vi "data insert core.vi"(8 "error in (no error)":errorcluster, 9 "column information":T1[](array[typedef]), 10 "data":variant[](array[variant]), 11 "table":string) -> (0 "error out":errorcluster)   [LabVIEW 2016, in "斯坦道原位多参数.lvlib"]
uses:
  <vilib>/addons/database/Auxilliary.llb/DB Tools Column Info.ctl
  <vilib>/addons/database/Auxilliary.llb/DB Tools DataTypes.ctl
  <vilib>/Utility/sysdir.llb/System Directory Type.ctl
  <vilib>/addons/database/Auxilliary.llb/DB Tools Transaction.ctl
  <vilib>/addons/database/Auxilliary.llb/DB Tools Isolation Level.ctl
  <vilib>/addons/database/Auxilliary.llb/DB Tools Parameter Info.ctl
  <vilib>/addons/database/Auxilliary.llb/DB Tools Parameter Dir.ctl
  <vilib>/addons/database/Connection.llb/DB Tools Open Connec (String).vi
  <vilib>/addons/database/Connection.llb/Conn Transaction.vi
  <vilib>/addons/database/Connection.llb/Conn Execute.vi
  <vilib>/addons/database/Recordset.llb/Rec Destroy - Connection.vi
  <vilib>/addons/database/Command.llb/Cmd Set Parameter Value (C).vi
  <vilib>/addons/database/Auxilliary.llb/DB Tools Format Datetime String (Time Stamp).vi
  <vilib>/addons/database/Command.llb/Cmd Execute.vi
  <vilib>/addons/database/Recordset.llb/Rec Destroy - Command.vi
  <vilib>/addons/database/Command.llb/Cmd Delete.vi
  <vilib>/addons/database/NI_Database_API.lvlib
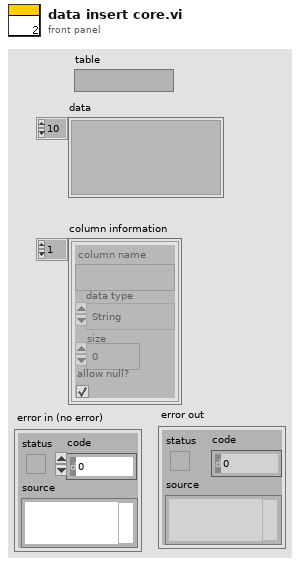
[diagram p1: front panel]
types:
  T1 = typedef "NI_Database_API.lvlib/DB Tools Column Info.ctl" = cluster{"column name":string, "data type":T2, "size":i32, "allow null?":bool}
  T2 = typedef "NI_Database_API.lvlib/DB Tools DataTypes.ctl" = enum16{"String", "Long (I32)", "Single (SGL)", "Double (DBL)", "Date/Time", "Binary"}
  T3 = typedef "NI_Database_API.lvlib/DB Tools Isolation Level.ctl" = enum16{"chaos", "read uncommitted", "read committed", "repeatable read", "serializable"}
  T4 = typedef "NI_Database_API.lvlib/DB Tools Transaction.ctl" = enum16{"begin", "commit", "rollback"}
  T5 = typedef "System Directory Type.ctl" = i32
  T6 = typedef "NI_Database_API.lvlib/Conn ObjectReference.ctl" = refnum<k1>
  T7 = typedef "NI_Database_API.lvlib/DB Tools Parameter Info.ctl" = cluster{"parameter name":string, "type":T2, "direction":T8, "value":variant}
  T8 = typedef "NI_Database_API.lvlib/DB Tools Parameter Dir.ctl" = enum32{"Input", "Output", "Input/Output", "Return Value"}
  T9 = typedef "NI_Database_API.lvlib/Rec ObjectReference.ctl" = refnum<k1>
  T10 = typedef "NI_Database_API.lvlib/Cmd ObjectReference.ctl" = refnum<k1>
  T11 = typedef "NI_Database_API.lvlib/Cmd-Rec Object Reference.ctl" = refnum<k1>
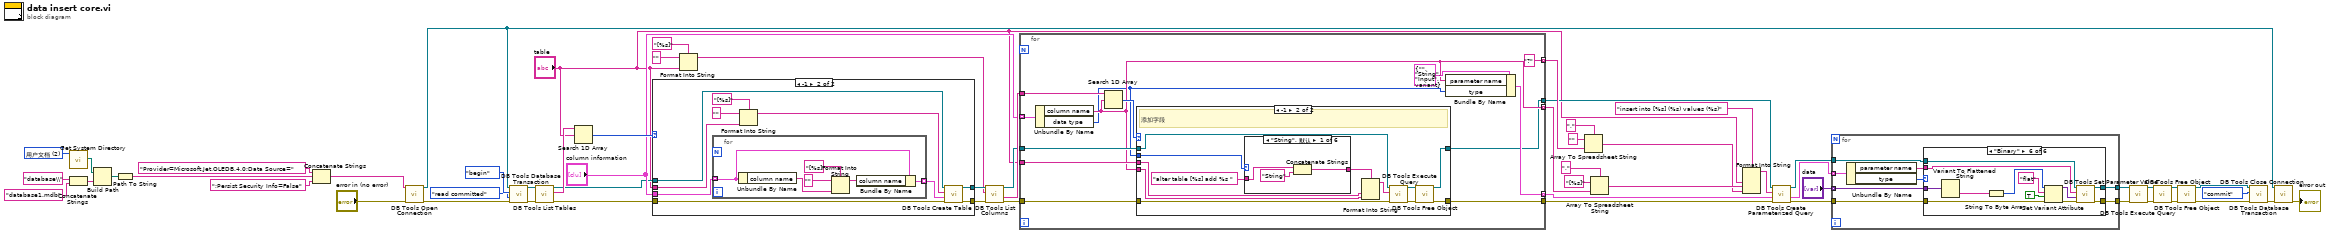
[diagram p0: block diagram]
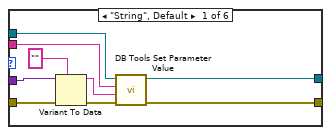
[diagram p2: hidden frame]
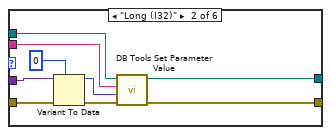
[diagram p3: hidden frame]
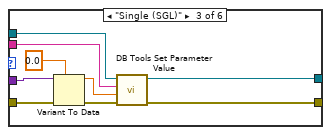
[diagram p4: hidden frame]
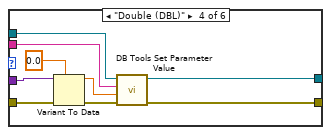
[diagram p5: hidden frame]
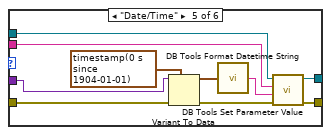
[diagram p6: hidden frame]
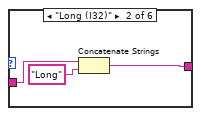
[diagram p8: hidden frame]
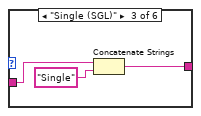
[diagram p9: hidden frame]
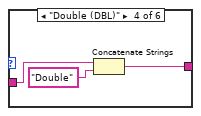
[diagram p10: hidden frame]
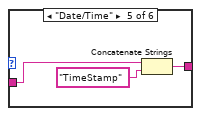
[diagram p11: hidden frame]
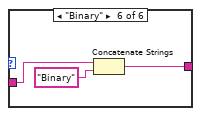
[diagram p12: hidden frame]
diagram:
  w59 = T5 2 items=["用户目录"=0, "用户桌面"=1, "用户文档"=2, "用户应用程序数据"=3, "用户设置"=4, "用户临时目录"=5, "公共文档"=6, "公共应用程序数据"=7, "公共设置"=8, "公共缓存"=13, "系统核心库"=9, "系统安装库"=10, "应用程序文件"=11, "启动盘根目录"=12] ("system directory type")
  n1 = call <vilib>:"Get System Directory.vi"("system directory type"=w59) -> ("system directory"=w57:path)  [unwired: 10 in]
  n2 = Concatenate Strings("database\\" ("condition"), "database1.mdb" ("database")) -> (w51:string)
  n3 = Build Path(base path=w57, name or relative path=w51) -> (appended path=w56:path)
  n4 = Path To String(path=w56) -> (string=w55:string)
  n5 = Concatenate Strings("Provider=Microsoft.Jet.OLEDB.4.0;Data Source=" ("condition"), w55, ";Persist Security Info=False" ("condition")) -> (w53:string)
  n6 = call-poly <vilib>:"DB Tools Open Connection.vi"("error in (no error)"="error in (no error)", "connection information"=w53) -> ("error out"=w13:errorcluster, "connection reference"=w5:T6)  [unwired: 6 in]
  n7 = call-poly <vilib>:"DB Tools Database Transaction.vi"("error in (no error)"=w13, "isolation level (chaos)"=DB_Tools_Isolation_Level."read committed", "operation (begin)"=DB_Tools_Transaction."begin", "connection reference"=w5) -> ("error out"=w12:errorcluster, "connection reference out"=w14:T6)  [unwired: 2 in]
  n8 = call <vilib>:"DB Tools List Tables.vi"("error in (no error)"=w12, "connection reference"=w14) -> ("error out"=w42:errorcluster, "tables"=w44:string[], "connection reference out"=w8:T6)  [unwired: 3 in]
  n9 = Search 1D Array(1D array=w44, element="table") -> (index of element=w43:i32)  [unwired: 1 in]
  n10 = case shown="-1" w43 {
    tunnel: w8 -> [w61 w71]
    tunnel: w42 -> [w60 w70]
    tunnel: "table" -> [_ w63]
    tunnel: "column information" -> [_ w67]
    tunnel: [w61 w69] -> w38
    tunnel: [w60 w68] -> w37
    frame 0, Default {
    }
    frame -1 {
      n11 = for {
        tunnel: w67 -> [w73] mode=indexing
        tunnel: [w72] -> w66 mode=indexing
        n12 = Unbundle By Name(w73) -> ("column name"=w77:string)
        n13 = Format Into String(format string="[%s]" ("格式字符串"), initial string="" ("初始字符串"), w77) -> (resulting string=w74:string)  [unwired: 1 in, 1 out]
        n14 = Bundle By Name(cluster=w73, "column name"=w74) -> (w72:T1)
      }
      n15 = Format Into String(format string="[%s]" ("格式字符串"), initial string="" ("初始字符串"), w63) -> (resulting string=w62:string)  [unwired: 1 in, 1 out]
      n16 = call <vilib>:"DB Tools Create Table.vi"("error in (no error)"=w70, "column information"=w66, "table"=w62, "connection reference"=w71) -> ("error out"=w68:errorcluster, "connection reference out"=w69:T6)  [unwired: 4 in]
    }
  }
  n17 = Format Into String(format string="[%s]" ("格式字符串"), initial string="" ("初始字符串"), "table") -> (resulting string=w1:string)  [unwired: 1 in, 1 out]
  n18 = call <vilib>:"DB Tools List Columns.vi"("error in (no error)"=w37, "table"=w1, "connection reference"=w38) -> ("error out"=w40:errorcluster, "columns"=w41:string[], "connection reference out"=w10:T6)  [unwired: 1 in, 1 out]
  n19 = for {
    tunnel: w10 -> [w88]
    tunnel: w41 -> [w90]
    tunnel: w40 -> [w87]
    tunnel: [w86] -> w36
    tunnel: "table" -> [w85]
    tunnel: "column information" -> [w84] mode=indexing
    tunnel: [w82] -> w35 mode=indexing
    tunnel: [w81] -> w29 mode=indexing
    tunnel: ["?"] -> w27 mode=indexing
    tunnel: [w78] -> w7
    n20 = Unbundle By Name(w84) -> ("column name"=w81:string, "data type"=w79:T2)
    n21 = Search 1D Array(1D array=w90, element=w81) -> (index of element=w89:i32)  [unwired: 1 in]
    n22 = case shown="-1" w89 {
      tunnel: [w92 w101] -> w86
      tunnel: w88 -> [w91 w100]
      tunnel: w81 -> [_ w99]
      tunnel: w87 -> [w92 w98]
      tunnel: w85 -> [_ w97]
      tunnel: w79 -> [_ w95]
      tunnel: [w91 w93] -> w78
      frame 0, Default {
      }
      frame -1 {
        # "添加字段"
        n23 = case shown="\"String\", 默认" w95 {
          tunnel: "alter table [%s] add %s " -> [w107 w110 w113 w116 w119 w122]
          tunnel: [w106 w109 w112 w115 w118 w121] -> w94
          frame "String", Default {
            n24 = Concatenate Strings(w107, "String" ("字符串")) -> (w106:string)
          }
          frame "Long (I32)" {
            n25 = Concatenate Strings(w110, "Long" ("字符串")) -> (w109:string)
          }
          frame "Single (SGL)" {
            n26 = Concatenate Strings(w113, "Single" ("字符串")) -> (w112:string)
          }
          frame "Double (DBL)" {
            n27 = Concatenate Strings(w116, "Double" ("字符串")) -> (w115:string)
          }
          frame "Date/Time" {
            n28 = Concatenate Strings(w119, "TimeStamp" ("字符串")) -> (w118:string)
          }
          frame "Binary" {
            n29 = Concatenate Strings(w122, "Binary" ("字符串")) -> (w121:string)
          }
        }
        n30 = Format Into String(format string=w94, w97, w99) -> (resulting string=w102:string)  [unwired: 2 in, 1 out]
        n31 = call-poly <vilib>:"DB Tools Execute Query.vi"("error in (no error)"=w98, "SQL query"=w102, "connection reference"=w100) -> ("error out"=w103:errorcluster, "recordset reference"=w104:T9)  [unwired: 5 in]
        n32 = call-poly <vilib>:"DB Tools Free Object.vi"("error in (no error)"=w103, "recordset reference"=w104) -> ("error out"=w101:errorcluster, "connection reference"=w93:T6)  [unwired: 8 in]
      }
    }
    n33 = Bundle By Name(cluster=T7 {"parameter name"="", "type"=enum."String", "direction"=enum."Input", "value"=variant} ("parameter information"), "parameter name"=w81, "type"=w79) -> (w82:T7)
  }
  n34 = Array To Spreadsheet String(delimiter (Tab)="," ("分隔符(Tab)"), array=w27, 3:"" ("格式字符串")) -> (spreadsheet string=w26:string)
  n35 = Array To Spreadsheet String(delimiter (Tab)="," ("分隔符(Tab)"), array=w29, 3:"[%s]" ("格式字符串")) -> (spreadsheet string=w28:string)
  n36 = Format Into String(format string="insert into [%s] (%s) values (%s)" ("格式字符串"), "table", w28, w26) -> (resulting string=w25:string)  [unwired: 2 in, 1 out]
  n37 = call <vilib>:"DB Tools Create Parameterized Query.vi"("error in (no error)"=w36, "parameters"=w35, "SQL query"=w25, "connection reference"=w7) -> ("error out"=w24:errorcluster, "parameters out"=w23:T7[], "command reference"=w9:T10)  [unwired: 3 in]
  n38 = for {
    tunnel: w9 -> [w127]
    tunnel: w24 -> [w125]
    tunnel: w23 -> [w130] mode=indexing
    tunnel: "data" -> [w128] mode=indexing
    tunnel: [w124] -> w6
    tunnel: [w123] -> w22
    n39 = Unbundle By Name(w130) -> ("parameter name"=w126:string, "type"=w129:T2)
    n40 = case shown="\"Binary\"" w129 {
      tunnel: w128 -> [w134 w142 w149 w159 w176 w180]
      tunnel: w127 -> [w137 w146 w153 w163 w174 w188]
      tunnel: w126 -> [w136 w145 w152 w158 w173 w187]
      tunnel: w125 -> [w131 w140 w150 w160 w171 w179]
      tunnel: [w133 w144 w154 w162 w170 w186] -> w124
      tunnel: [w132 w143 w151 w161 w169 w185] -> w123
      frame "String", Default {
        n41 = Variant To Data(error in=w131, type="", Variant=w134) -> (data=w135:string, error out=w139:errorcluster)
        n42 = call-poly <vilib>:"DB Tools Set Parameter Value.vi"("error in (no error)"=w139, "value"=w135, "parameter index"=w136, "command reference"=w137) -> ("error out"=w132:errorcluster, "command reference out"=w133:T10)  [unwired: 4 in]
      }
      frame "Long (I32)" {
        n43 = Variant To Data(error in=w140, type=0, Variant=w142) -> (data=w147:i32, error out=w148:errorcluster)
        n44 = call-poly <vilib>:"DB Tools Set Parameter Value.vi"("error in (no error)"=w148, "value"=w147, "parameter index"=w145, "command reference"=w146) -> ("error out"=w143:errorcluster, "command reference out"=w144:T10)  [unwired: 4 in]
      }
      frame "Single (SGL)" {
        n45 = Variant To Data(error in=w150, type=sgl 0.0, Variant=w149) -> (data=w156:sgl, error out=w157:errorcluster)
        n46 = call-poly <vilib>:"DB Tools Set Parameter Value.vi"("error in (no error)"=w157, "value"=w156, "parameter index"=w152, "command reference"=w153) -> ("error out"=w151:errorcluster, "command reference out"=w154:T10)  [unwired: 4 in]
      }
      frame "Double (DBL)" {
        n47 = Variant To Data(error in=w160, type=0.0, Variant=w159) -> (data=w165:dbl, error out=w166:errorcluster)
        n48 = call-poly <vilib>:"DB Tools Set Parameter Value.vi"("error in (no error)"=w166, "value"=w165, "parameter index"=w158, "command reference"=w163) -> ("error out"=w161:errorcluster, "command reference out"=w162:T10)  [unwired: 4 in]
      }
      frame "Date/Time" {
        n49 = Variant To Data(error in=w171, type=timestamp(0 s since 1904-01-01) ("时间标识"), Variant=w176) -> (data=w168:timestamp, error out=w172:errorcluster)
        n50 = call-poly <vilib>:"DB Tools Format Datetime String.vi"("time stamp"=w168) -> ("date/time string"=w167:string)
        n51 = call-poly <vilib>:"DB Tools Set Parameter Value.vi"("error in (no error)"=w172, "value"=w167, "parameter index"=w173, "command reference"=w174) -> ("error out"=w169:errorcluster, "command reference out"=w170:T10)  [unwired: 4 in]
      }
      frame "Binary" {
        n52 = Variant To Flattened String(Variant=w180) -> (data string=w181:string)  [unwired: 1 out]
        n53 = String To Byte Array(string=w181) -> (unsigned byte array=w184:u8[])
        n54 = Set Variant Attribute(Variant=w184, name="flat", value=TRUE, error in=w179) -> (Variant out=w177:variant, error out=w178:errorcluster)  [unwired: 1 out]
        n55 = call-poly <vilib>:"DB Tools Set Parameter Value.vi"("error in (no error)"=w178, "value"=w177, "parameter index"=w187, "command reference"=w188) -> ("error out"=w185:errorcluster, "command reference out"=w186:T10)  [unwired: 4 in]
      }
    }
  }
  n56 = call-poly <vilib>:"DB Tools Execute Query.vi"("error in (no error)"=w22, "command reference"=w6) -> ("error out"=w20:errorcluster, "command-recordset reference"=w21:T11)  [unwired: 6 in]
  n57 = call-poly <vilib>:"DB Tools Free Object.vi"("error in (no error)"=w20, "command-recordset reference"=w21) -> ("error out"=w18:errorcluster, "command reference"=w19:T10)  [unwired: 8 in]
  n58 = call-poly <vilib>:"DB Tools Free Object.vi"("error in (no error)"=w18, "command reference"=w19) -> ("error out"=w15:errorcluster, "connection reference"=w16:T6)  [unwired: 8 in]
  n59 = call-poly <vilib>:"DB Tools Database Transaction.vi"("error in (no error)"=w15, "operation (begin)"=DB_Tools_Transaction."commit", "connection reference"=w16) -> ("error out"=w17:errorcluster)  [unwired: 3 in, 1 out]
  n60 = call <vilib>:"DB Tools Close Connection.vi"("error in (no error)"=w17, "connection reference"=w5) -> ("error out"=→"error out":errorcluster)  [unwired: 5 in]
